vi "Sandbox 8 - Get LLB version.vi"() -> ()   [LabVIEW 2022 SP3]
uses:
  <vilib>/Utility/libraryn.llb/Librarian File Info Out.ctl
  <vilib>/Utility/libraryn.llb/Librarian File List.ctl
  <userlib>/_OpenG.lib/file/file.llb/File Info Record__ogtk.ctl
  4a639bdb-a42e-4fa2-ab26-023ca618b39d.vi
  <vilib>/Comparison/Less/Less Functor/Less Functor.lvclass
panel:
  out "VI's contained inside LLB":string[](array[string])
  out "file info":T1={"type"="????", "creator"="????", "permissions"=438, "data size"=5687, "res size"=0, "creation date"=3188231670, "modification date"=3188232972, "bFolder"=FALSE, "bInvisible"=FALSE, "location"={"vertical"=0, "horizontal"=0}, "owner"="", "group"=""} {"modification date" format="%<%H:%M:%S\n%m/%d/%Y>T"; "creation date" format="%<%H:%M:%S\n%m/%d/%Y>T"; "permissions" format="%.0x"}
  out "size(s)":i32
  out "file list":T2 {"LV version" format="%.0x"}
  out "file information":T3 {"LV version" format="%.0x"}
  out "error out":errorcluster
  out "file information out":T3 {"LV version" format="%.0x"}
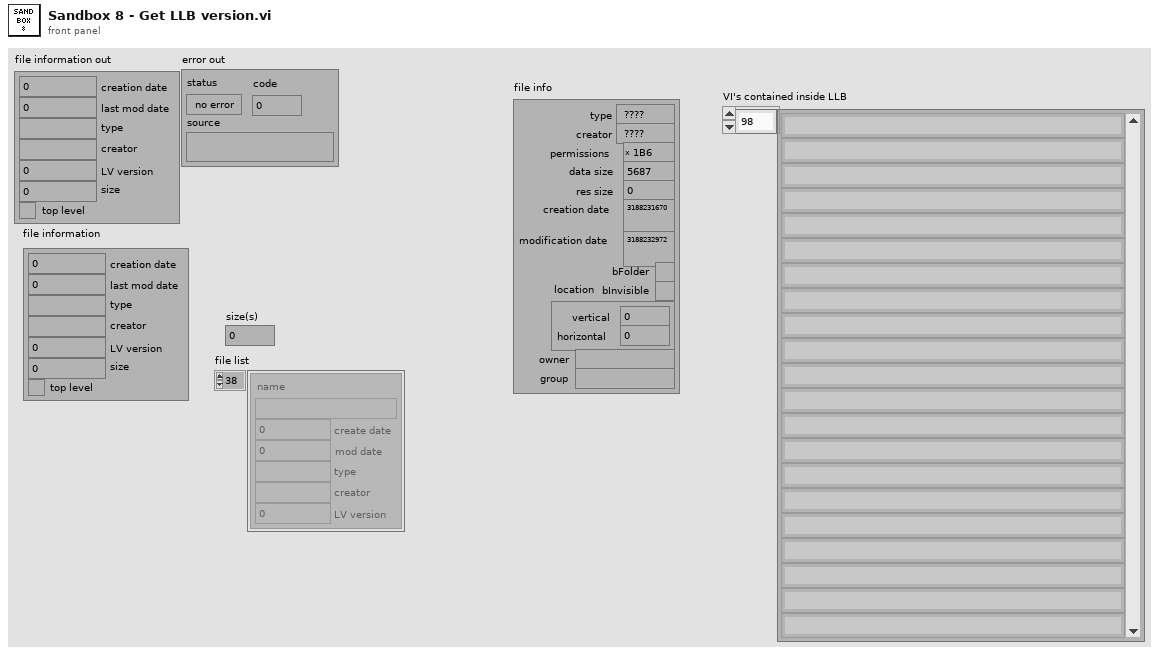
[diagram p1: front panel]
types:
  T1 = typedef "File Info Record__ogtk.ctl" = cluster{"type":string, "creator":string, "permissions":i32, "data size":i32, "res size":i32, "creation date":u32, "modification date":u32, "bFolder":bool, "bInvisible":bool, "location":cluster{"vertical":i16, "horizontal":i16}, "owner":string, "group":string}
  T2 = typedef "Librarian File List.ctl" = cluster{"name":string, "create date":u32, "mod date":u32, "type":string, "creator":string, "LV version":i32}[]
  T3 = typedef "Librarian File Info Out.ctl" = cluster{"creation date":u32, "last mod date":u32, "type":string, "creator":string, "LV version":i32, "size":i32, "top level":bool}
  T4 = enum16{"get library file information", "set library file information", "copy file", "move file", "delete file", "get library list"}
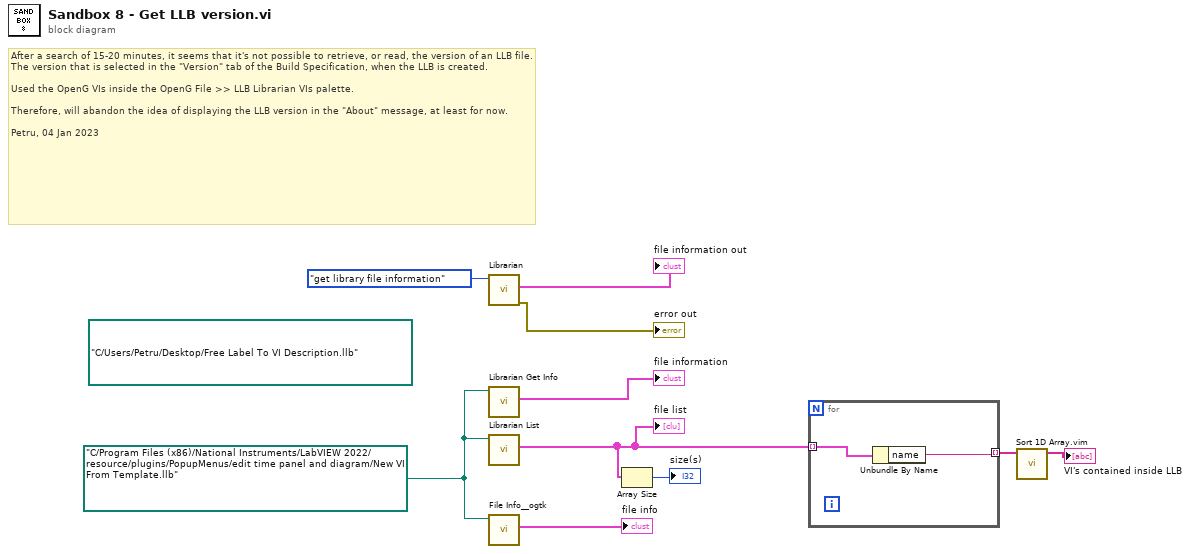
[diagram p0: block diagram]
diagram:
  w4 = path "C:/Program Files (x86)/National Instruments/LabVIEW 2022/resource/plugins/PopupMenus/edit time panel and diagram/New VI From Template.llb"
  (unwired) path "C:/Users/Petru/Desktop/Free Label To VI Description.llb"
  # "After a search of 15-20 minutes, it seems that it's not possible to retrieve, or read, the version of an LLB file. The version that is selected in the \"Version\" tab of the Build Specification, when the LLB is created. \n\nUsed the OpenG VIs inside the OpenG File >> LLB Librarian VIs palette.\n\nTherefore, will abandon the idea of displaying the LLB version in the \"About\" message, at least for now.\n\nPetru, 04 Jan 2023"
  n1 = call <vilib>:"Librarian.vi"("operation"=T4."get library file information") -> ("error out"=→"error out":errorcluster, "file information out"=→"file information out":T3)  [unwired: 8 in, 1 out]
  n2 = call <vilib>:"Librarian Get Info.vi"("path"=w4) -> ("file information"=→"file information":T3)  [unwired: 8 in, 2 out]
  n3 = call <vilib>:"Librarian List.vi"("path"=w4) -> ("file list"=w3:T2)  [unwired: 9 in, 1 out]
  "file list" <- w3
  n4 = call <userlib>:"File Info__ogtk.vi"("file"=w4) -> ("file info"=→"file info":T1)  [unwired: 5 in, 2 out]
  n5 = Array Size(array=w3) -> (size(s)=→"size(s)":i32)
  n6 = for {
    tunnel: w3 -> [w12] mode=indexing
    tunnel: [w11] -> w2 mode=indexing
    n7 = Unbundle By Name(w12) -> ("name"=w11:string)
  }
  n8 = call "Sort 1D Array.vim"("unsorted array"=w2) -> ("sorted array"=→"VI's contained inside LLB":string[])  [unwired: 10 in]
